vi "WSVCAP SHL Host LL RFFE Convert Channel Bytes to Bit Array.vi"(0 "RFFE Data [DUT Ordered]":u8[][](array[numeric]) format="%02x", 7 "Cycle CMD Lengths Out (bits)":u8[](array[numeric]), 9 "Cycle CMD Delay Out (ticks)":u32[](array[numeric])) -> (4 "Write Data":u64[](array[numeric]) format="%016x")   [LabVIEW 2012]
panel:
  # "D0"
  # "D4"
  # "D8"
  # "D12"
  # "D16"
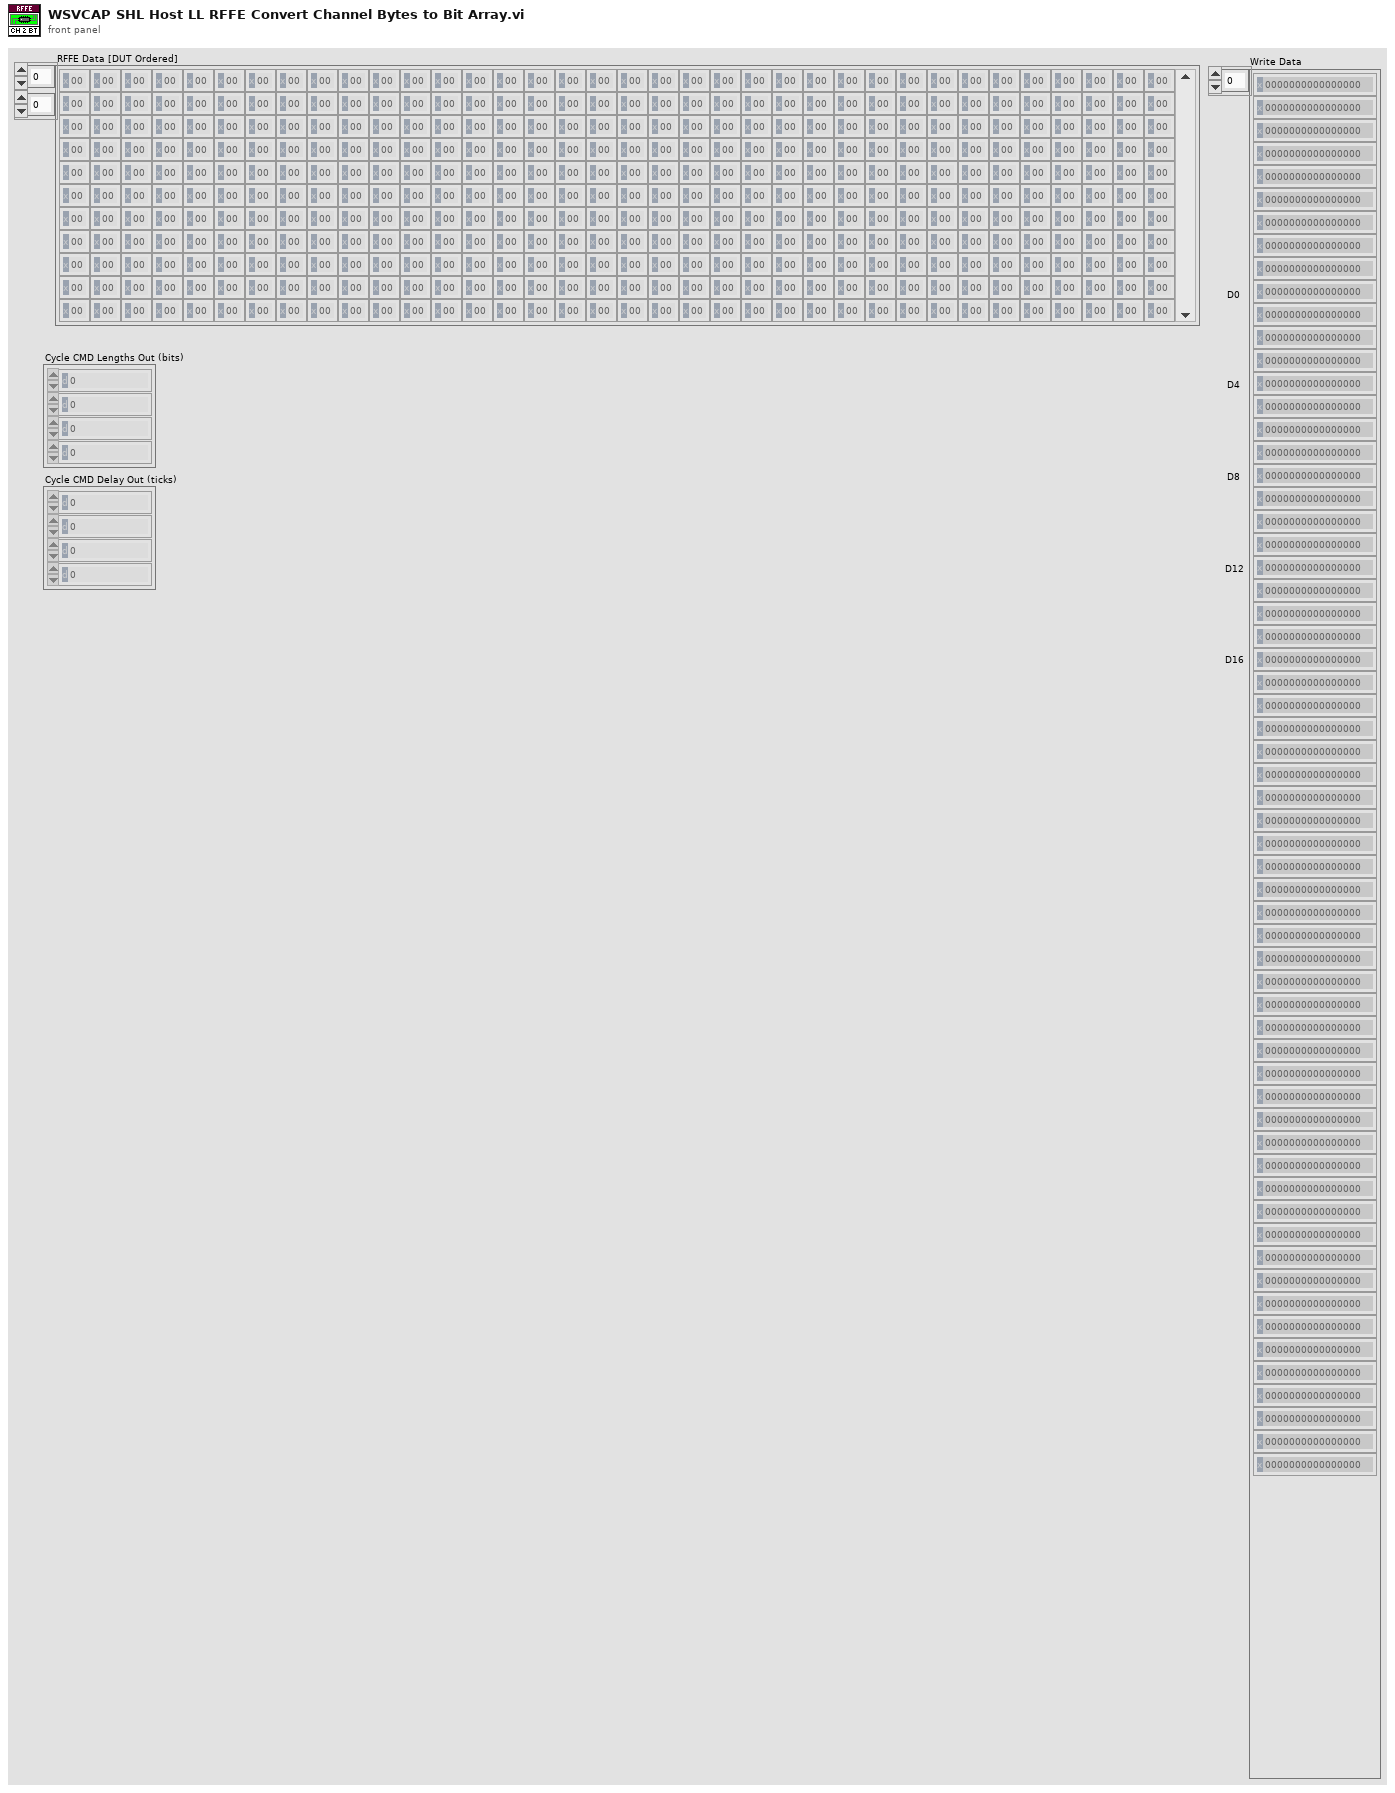
[diagram p1: front panel]
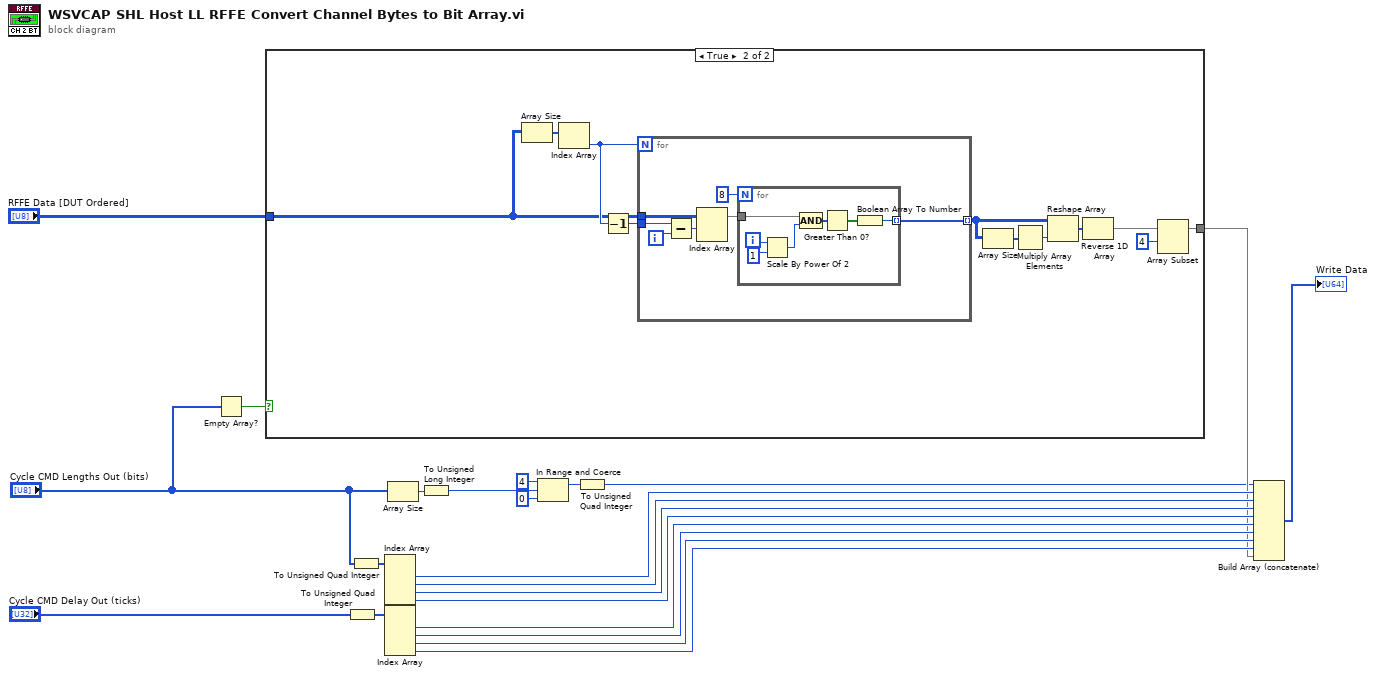
[diagram p0: block diagram]
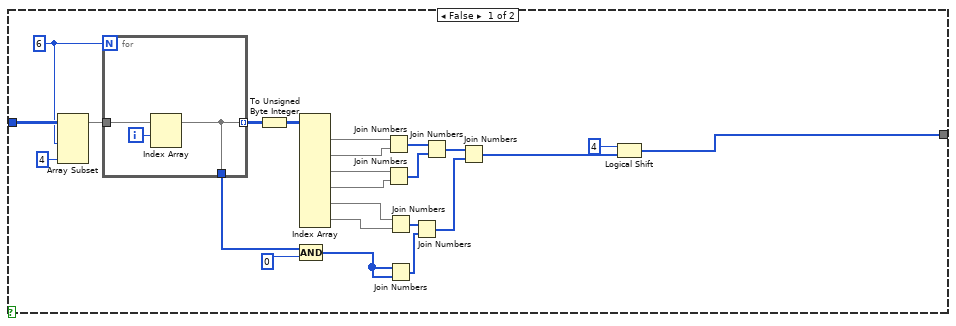
[diagram p2: hidden frame]
diagram:
  n1 = Empty Array?(array="Cycle CMD Lengths Out (bits)") -> (empty?=w3:bool)
  n2 = case shown="True" w3 {
    tunnel: "RFFE Data [DUT Ordered]" -> [w33 w51]
    tunnel: [w24 w53] -> w5
    frame False {
      w31 = 6
      n3 = Array Subset(array=w33, length (row)=w31, length (col)=4 ("length")) -> (w32:u8[][])  [unwired: 2 in]
      n4 = for {
        N: w31 -> [_]
        tunnel: w32 -> [w49]
        tunnel: [w47] -> w34 mode=indexing
        tunnel: [w47] -> w29
        i -> [w48]
        n5 = Index Array(array=w49, index (row)=w48) -> (element=w47:u8[])  [unwired: 1 in]
      }
      n6 = To Unsigned Byte Integer(number=w34) -> (unsigned 8bit integer=w39:u8[][])
      n7 = Index Array(array=w39) -> (element #1=w46:u8[], element #2=w45:u8[], element #3=w44:u8[], element #4=w43:u8[], element #5=w38:u8[], element #6=w26:u8[])  [unwired: 12 in]
      n8 = Compound Arithmetic op=AND(w29, u8 0 ("Read Data")) -> (w28:u8[])
      n9 = Join Numbers(hi=w46, lo=w45) -> ((hi.lo)=w42:u16[])
      n10 = Join Numbers(hi=w44, lo=w43) -> ((hi.lo)=w41:u16[])
      n11 = Join Numbers(hi=w38, lo=w26) -> ((hi.lo)=w37:u16[])
      n12 = Join Numbers(hi=w28, lo=w28) -> ((hi.lo)=w36:u16[])
      n13 = Join Numbers(hi=w37, lo=w36) -> ((hi.lo)=w35:u32[])
      n14 = Join Numbers(hi=w42, lo=w41) -> ((hi.lo)=w40:u32[])
      n15 = Join Numbers(hi=w40, lo=w35) -> ((hi.lo)=w25:u64[])
      n16 = Logical Shift(y=i16 4, x=w25) -> (x << y=w24:u64[])
    }
    frame True {
      n17 = Array Size(array=w51) -> (size(s)=w57:i32[])
      n18 = Index Array(array=w57) -> (element=w55:i32)  [unwired: 1 in]
      n19 = Decrement(x=w55) -> (x-1=w54:i32)
      n20 = for {
        N: w55 -> [_]
        tunnel: w51 -> [w65]
        tunnel: [w66] -> w60 mode=indexing
        tunnel: w54 -> [w61]
        i -> [w63]
        n21 = Subtract(x=w61, y=w63) -> (x-y=w62:i32)
        n22 = Index Array(array=w65, index (row)=w62) -> (element=w64:u8[])  [unwired: 1 in]
        n23 = for {
          N: 8 -> [_]
          tunnel: w64 -> [w70]
          tunnel: [w69] -> w66 mode=indexing
          i -> [w72]
          n24 = Scale By Power Of 2(n=w72, x=u8 1) -> (x*2^n=w73:u8)
          n25 = Compound Arithmetic op=AND(w70, w73) -> (w74:u8[])
          n26 = Greater Than 0?(x=w74) -> (x > 0?=w68:bool[])
          n27 = Boolean Array To Number(Boolean array=w68) -> (number=w69:u64)
        }
      }
      n28 = Array Size(array=w60) -> (size(s)=w59:i32[])
      n29 = Multiply Array Elements(1:w59) -> (0:w58:i32)
      n30 = Reshape Array(w60, w58) -> (w56:u64[])
      n31 = Reverse 1D Array(array=w56) -> (reversed array=w50:u64[])
      n32 = Array Subset(array=w50, index=4) -> (w53:u64[])  [unwired: 1 in]
    }
  }
  n33 = To Unsigned Quad Integer(1:"Cycle CMD Delay Out (ticks)") -> (0:w2:u64[])
  n34 = To Unsigned Quad Integer(1:"Cycle CMD Lengths Out (bits)") -> (0:w14:u64[])
  n35 = Index Array(array=w14) -> (element #1=w16:u64, element #2=w15:u64, element #3=w13:u64, element #4=w12:u64)  [unwired: 4 in]
  n36 = Index Array(array=w2) -> (element #1=w11:u64, element #2=w10:u64, element #3=w9:u64, element #4=w8:u64)  [unwired: 4 in]
  n37 = Array Size(array="Cycle CMD Lengths Out (bits)") -> (size(s)=w21:i32)
  n38 = To Unsigned Long Integer(number=w21) -> (unsigned 32bit integer=w6:u32)
  n39 = In Range and Coerce(upper limit=u32 4, x=w6, lower limit=u32 0) -> (coerced(x)=w18:u32)  [unwired: 1 out]
  n40 = To Unsigned Quad Integer(1:w18) -> (0:w1:u64)
  n41 = Build Array (concatenate)(w1, w16, w15, w13, w12, w11, w10, w9, w8, w5) -> (→"Write Data":u64[])
